vi "LIA Scale Acquired Data NI 5783.vi"(6 "range (V)":dbl=2.0, 9 "Sample Rate":dbl=100000000.0, 10 "Number of Bits":i16=14, 11 "Data In":i16[](array[numeric])) -> (3 "Data":waveform(dbl)[](array[waveform]))   [LabVIEW 2017]
doc: "This VI scales the raw data returned by the adapter module from ADC codes to volts. It also stores the data in a waveform data type and sets the sample rate for the waveform."
panel:
  out "x/y":dbl
  # "Refer to the Block Diagram of this VI for execution comments."
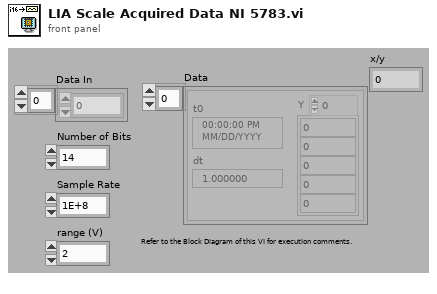
[diagram p1: front panel]
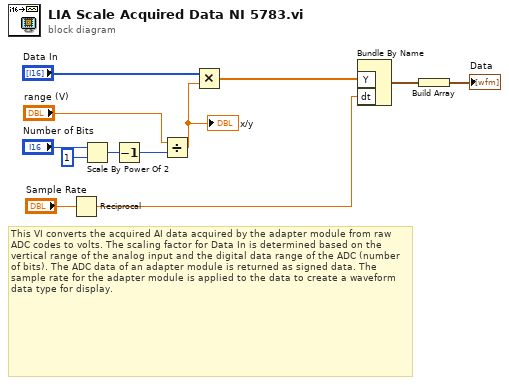
[diagram p0: block diagram]
diagram:
  # "This VI converts the acquired AI data acquired by the adapter module from raw ADC codes to volts. The scaling factor for Data In is determined based on the vertical range of the analog input and the digital data range of the ADC (number of bits). The ADC data of an adapter module is returned as signed data. The sample rate for the adapter module is applied to the data to create a waveform data type for display."
  n1 = Reciprocal(x="Sample Rate") -> (1/x=w10:dbl)
  n2 = Scale By Power Of 2(n="Number of Bits", x=1) -> (x*2^n=w11:i32)
  n3 = Decrement(x=w11) -> (x-1=w6:i32)
  n4 = Divide(x="range (V)", y=w6) -> (x/y=w4:dbl)
  "x/y" <- w4
  n5 = Multiply(x="Data In", y=w4) -> (x*y=w2:dbl[])
  n6 = Bundle By Name("Y"=w2, "dt"=w10) -> (w3:waveform(dbl))  [unwired: 1 out]
  n7 = Build Array(w3) -> (→"Data":waveform(dbl)[])
